vi "Elevator - Send Command.vi"(8 "error in (no error)":errorcluster, 9 "Variant":variant, 10 "Elevator Commands":T1, 11 "View Model":T2) -> (0 "error out":errorcluster, 3 "View Model":T2)   [LabVIEW 2017]
doc: "Sends commands to elevator controller"
uses:
  View Model/Controls/View Model.ctl
  Error Handler/Controls/Error Model.ctl
  Error Handler/Controls/Error EventData.ctl
  Error Handler/Controls/Error Type.ctl
  Controls/Elevator Model.ctl
  Controls/Elevator Overhead.ctl
  Controls/Elevator States.ctl
  Controls/Elevator Location.ctl
  Controls/Elevator Command Event.ctl
  Controls/Elevator Commands.ctl
  Configuration/Controls/Configuration Model.ctl
  Configuration/Controls/Configuration Data.ctl
  View Model/Controls/Shared Model.ctl
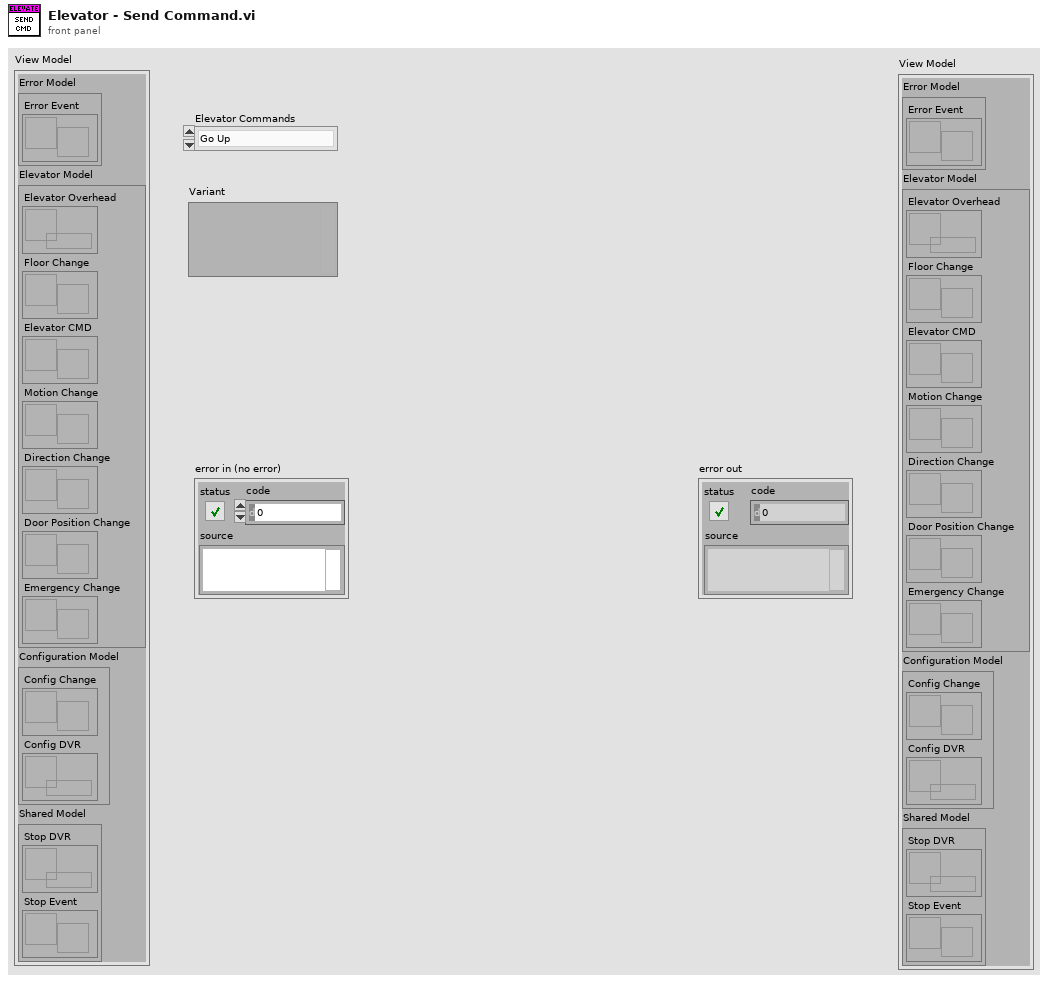
[diagram p1: front panel]
types:
  T1 = typedef "Elevator Commands.ctl" = enum16{"Go Up", "Go Down", "Go to Floor", "Emergency", "Open Doors", "Close Doors"}
  T2 = typedef "View Model.ctl" = cluster{"Error Model":T3, "Elevator Model":T4, "Configuration Model":T5, "Shared Model":T6}
  T3 = typedef "Error Model.ctl" = cluster{"Error Event":refnum<user-event>}
  T4 = typedef "Elevator Model.ctl" = cluster{"Elevator Overhead":refnum<data-value>, "Floor Change":refnum<user-event>, "Elevator CMD":refnum<user-event>, "Motion Change":refnum<user-event>, "Direction Change":refnum<user-event>, "Door Position Change":refnum<user-event>, "Emergency Change":refnum<user-event>}
  T5 = typedef "Configuration Model.ctl" = cluster{"Config Change":refnum<user-event>, "Config DVR":refnum<data-value>}
  T6 = typedef "Shared Model.ctl" = cluster{"Stop DVR":refnum<data-value>, "Stop Event":refnum<user-event>}
  T7 = typedef "Elevator Command Event.ctl" = cluster{"Elevator Commands":T1, "Variant":variant}
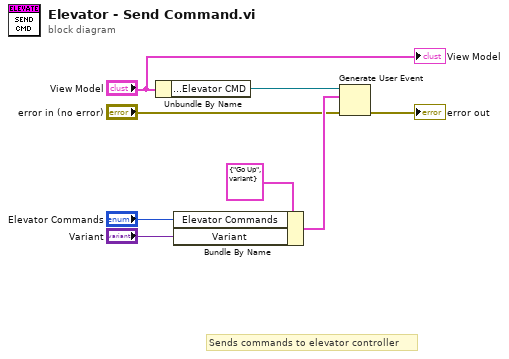
[diagram p0: block diagram]
diagram:
  # "Sends commands to elevator controller"
  n1 = Unbundle By Name("View Model") -> ("Elevator Model.Elevator CMD"=w8:refnum<user-event>)
  n2 = Bundle By Name(cluster=T7 {"Elevator Commands"=enum."Go Up", "Variant"=variant} ("Elevator CMD Event"), "Elevator Commands"="Elevator Commands", "Variant"="Variant") -> (w4:T7)
  n3 = Generate User Event(user event=w8, event data cluster=w4, error in="error in (no error)") -> (error out=→"error out":errorcluster)  [unwired: 1 in, 1 out]
  "View Model" <- "View Model"
